vi "Main_19a.vi"() -> ()   [LabVIEW 2023]
uses:
  Cluster_Rule.ctl
  ENUM_Compare.ctl
  ENUM_Value Type.ctl
  <vilib>/Utility/error.llb/Trim Whitespace One-Sided.vi
panel:
  out "Accept Array":i32[][](array[numeric])
  out "Number Array":i32[][](array[numeric])
  out "Map":map{string, T1[]}(c390)
  out "Answer":i32
  in  "Puzzle":string="jtx{s<3181:R,R}\nrkd{s>2386:tdr,R}\nsvj{x>1520:A,A}\nvkv{x<3627:A,x>3794:A,A}\nksz{m<1450:R,a<2837:R,a<2928:R,A}\nfp{x<1293:sjt,bv}\njq{m>1493:R,m>1377:A,m<1344:R,R}\ngts{m<3166:R,A}\nxxr{s<231:R,x<3055:R,R}\nrz{a<2982:A,m<1763:R,x>1878:A,A}\nkq{s<2900:R,s>3591:A,R}\ntmg{s<1500:A,x>2504:R,a<1166:A,R}\ndvn{s<1632:R,A}\nznj{m>1884:A,R}\ndb{m<1554:cg,m>3173:R,x<1203:A,xsm}\nchr{a<682:R,x>3120:R,m>2313:A,R}\npd{x<1433:kp,a<2715:fjd,xtx}\nqkd{s<666:R,R}\nrbf{x>2541:R,R}\ngx{s>1347:A,m<812:gxz,s>1079:tpg,lt}\nfqb{x<1290:A,R}\njf{x<1340:A,s>2972:dq,x>1378:bqh,jps}\nsr{m>776:A,A}\nvs{s<1377:R,R}\nvx{x>1237:R,A}\ndz{m<192:A,m<271:A,R}\nmhr{m<2568:R,m<3466:R,a>3791:A,R}\nvv{m<3559:A,s>3108:R,R}\npsk{a>2830:A,a<2278:A,A}\ngvv{a>2993:A,a>2553:A,R}\ngsx{x<2656:A,A}\njps{a<1216:A,R}\nlt{s<967:A,A}\nng{s<3259:R,s<3674:R,A}\nzd{s>2267:R,R}\nks{a>1951:bg,m<1522:gpf,gj}\nprk{m<2242:R,s>56:R,R}\nnr{x>3432:R,sg}\nfkd{s>2014:mxf,sps}\ntk{x<1133:jzj,vq}\nsgl{a<1237:R,A}\nsmg{x<2071:R,m<387:R,A}\nqd{s<3197:sl,x>1479:lqs,m>1300:rrp,gm}\ntr{s<1306:R,x>1183:A,A}\nbxh{a>1123:fpp,R}\nhjp{a>2545:nb,a>2381:qx,m>2463:nn,bt}\nzg{s<1932:smc,m<1443:rq,jf}\nnnq{m>3341:lx,s<2737:A,a<3408:A,R}\nlx{s>3219:A,a>2886:A,m<3691:A,R}\nstl{s<2701:R,m>3442:A,s<3282:A,A}\ngsp{m<619:R,s<529:R,A}\nfkk{x<3359:svx,sp}\ndsk{x<1499:kn,xj}\njmx{m<1426:zq,fvz}\nst{s>2257:slt,rvv}\nprm{a<470:A,tts}\nfkj{x<2514:R,x>2784:R,a>2830:R,qft}\nbh{m<1740:mmf,a>503:zn,s>1702:vfp,fft}\nrv{m<2642:A,sfv}\nqk{s<1846:A,A}\nnqr{a>786:ssx,qbh}\nkng{a<3059:A,a<3463:A,a<3661:A,A}\ntcd{m<3753:R,a<2566:pq,m<3792:R,hsq}\nrhc{x>1415:mzt,x>1395:qp,x>1386:rk,nnq}\nhn{x>3532:A,a>1227:R,a>1109:A,R}\nbtd{s<2462:ftz,A}\nxv{s>1573:pv,m>730:pn,s<1201:vtz,fjk}\nsm{a>787:R,R}\nmqz{m<645:R,m<682:A,A}\nrvv{m<867:vkv,a>556:R,mx}\nfft{x>581:jb,a<314:R,R}\ntxz{s<1338:R,x>2633:A,m<1168:A,A}\npcq{x<1531:A,R}\nkvj{s<2721:A,x>2637:A,R}\nkfj{x<1129:kz,s>1501:zfm,pk}\nrd{m<3742:A,A}\nqft{x<2653:A,s>1281:A,A}\nzzr{a<3875:R,m>249:A,a<3917:R,A}\nnh{a>3744:zcn,gxg}\nfsp{m>3306:R,R}\nrt{m<310:zlk,qgj}\nmpb{m>2954:R,R}\nqgj{s>1083:R,m<502:A,s<949:A,A}\nhq{x<1527:dfg,m>3017:jvm,a>947:jts,gqf}\nbfc{x>1423:R,a<2789:A,A}\nbnv{a>900:R,A}\ntdr{a>518:R,m>657:A,x>2576:R,R}\njmm{a<3410:mq,fv}\nqjr{a>2534:R,s<1365:A,m<261:A,R}\nin{x<1624:zsf,ks}\njgs{m<702:R,A}\nqg{a<1733:A,R}\npv{x<1559:hnp,x>1588:gbv,R}\nrpx{m<2361:zv,A}\nbzm{x<1510:rhc,x<1580:lct,m>3357:rrj,zld}\ndnf{x>2931:xkp,s>1747:A,s<858:qhb,zf}\nsk{x>3528:A,x<3113:bnx,psk}\nxgt{s>2544:vn,sft}\nkjv{s>1334:gsh,a>95:rbf,a>50:bmf,trd}\npvt{s>2784:A,s<2303:qk,a<1589:A,R}\nnv{a>3108:R,x>1923:R,s>652:A,A}\nnlg{m>383:A,s>1520:A,s>749:R,R}\nlk{a<2425:R,s>598:R,a>2517:R,A}\nnt{m>1682:R,m>999:A,m>428:A,A}\nrmp{m>2634:R,s<317:nt,lk}\nfs{m<2408:A,x<1842:R,R}\nsjt{x<1133:nqr,vt}\ntbk{m<2779:R,a>3554:R,a>3415:A,R}\njr{m>3312:A,R}\nbmf{s<509:xxs,a<68:qxr,R}\nxz{s<1845:A,x<1392:A,A}\ntpn{m>2419:A,x>2999:A,s<2347:A,R}\nfcg{a<196:A,m>1248:nbt,a>276:R,R}\nkv{x>1467:R,m>891:R,s>2429:A,A}\nrq{m>570:bft,x<1349:R,m<215:R,A}\ncpr{s>140:cdl,m<2079:znj,prk}\nfc{a<3507:R,x<1454:A,s<1296:A,A}\nkfs{x<2459:R,A}\nvr{m<3596:A,a<2837:R,A}\nvg{a>3513:xl,x<569:sr,x>740:bp,qxs}\nmzc{m<3026:R,a>1169:A,A}\njhk{m<3520:A,m<3692:A,a<701:R,A}\nqx{s<1241:A,A}\nbv{x<1412:zg,m<1721:hh,hq}\npj{s>3641:A,x>1535:mj,m<1145:A,jxb}\nsvx{x<3194:A,m<1734:gsp,m<2937:zk,kng}\nkp{x<1404:jj,m>1015:R,x>1415:bfc,A}\ncxh{m>619:R,m>536:A,R}\nffj{x<2728:R,s<231:A,R}\nfh{m<1629:A,a<1260:A,A}\ntrd{a>29:qc,A}\nhj{a<706:kvj,s<3197:grd,a>1057:mzc,gsx}\nqcx{a<265:R,R}\nbhz{x<1415:R,A}\nccq{a<3195:mtr,a<3700:jzv,x>1501:xv,tj}\nqpn{s>499:vpz,a>804:qsc,lsm}\njk{x<3497:R,x>3734:A,A}\nbz{x>568:A,a<773:A,R}\nhkv{a<1753:R,x<2544:A,a>1849:R,ps}\ngj{m>2405:fkd,s>1405:pf,qpn}\nlg{a<1611:rlx,a<1731:fps,A}\nln{a<1637:R,s<3175:A,A}\nshk{a<1729:htt,m>1833:R,A}\nsct{m>1497:A,R}\nrnj{a>2878:R,m>1475:R,a<2792:R,A}\nqp{a<3308:R,m>3268:vv,A}\nvq{s<2622:R,R}\nnbt{s<1656:A,m<1413:R,m>1485:A,A}\nbdm{x<2476:gv,x>2650:vhv,kh}\nbjh{x<2660:R,A}\nfnx{a<3874:A,A}\nqzt{s>3620:A,A}\nft{a<1286:A,m>1846:R,R}\ncx{a>2841:A,m<425:qjr,s>1229:qm,R}\nrrj{m<3695:nm,m>3867:sz,a>3080:cd,tcd}\nghj{s<2416:A,m<2698:R,R}\nxm{a<3638:pcq,m>2433:pnx,tsc}\nhkg{a<1186:A,R}\nts{s>905:A,m<299:R,R}\ndbf{m<1691:sct,s<3740:mnr,A}\nssq{s>3183:A,m<2388:A,A}\nbd{s>291:jbg,s<217:R,s<250:ffj,vl}\ndq{a<1136:R,R}\nrpf{s>2706:ll,x<2910:ghj,A}\nqxr{s<877:A,A}\nlct{s>3272:kx,hcp}\nbbc{a<3031:R,x<1554:A,R}\nzlk{m>176:R,A}\nlh{a<3217:fld,x<504:jr,rgg}\nzct{x>2738:sk,x>2209:bdm,gdm}\ndj{x>1137:A,a>2578:A,R}\ngc{a>2861:R,a<2739:A,A}\nlhn{s>2175:jz,m>1213:hcq,lxj}\nqm{x<1501:R,s>1724:R,A}\nbnx{s>3556:R,x<2924:A,a>2767:A,R}\nzr{s<2643:A,ms}\nsmc{x<1354:R,x>1374:R,s>1279:fh,cxb}\njvm{s>1609:zmn,a<1172:jhk,cxl}\nsz{s>3310:A,R}\nbxf{a>2995:A,rnj}\nqn{x>1577:A,R}\nrm{x>3502:sm,x<3166:rzf,R}\nzzd{a<2945:A,s<530:A,a<3360:A,A}\nns{x<1515:A,a<2501:A,R}\nrnb{s<1360:A,m>2498:R,s<1805:R,A}\nsrj{x>1408:R,R}\njzv{m>750:ltd,s<1511:rt,tcc}\ngps{a>3444:A,x>1039:R,x<989:R,A}\ncmr{x<2302:A,R}\nmgq{a>3431:A,m<2513:R,R}\nzps{m<2495:R,x>1582:A,a>3314:R,A}\nxj{s<2468:A,x>1516:A,a>3292:A,A}\nhfv{a>2835:phz,x<1072:jc,dj}\nvmf{a<2879:qdv,m<1506:xsn,x>2082:rr,xdq}\nndj{m>605:A,a>1367:R,A}\nsd{x>1431:A,a<3334:A,s>3667:A,A}\nfjt{a<2589:R,A}\nslp{x<583:A,A}\njfx{s>639:R,s>549:R,zc}\nzrc{m<2490:A,fsp}\nsqf{s>3315:A,m<2054:A,R}\nhlm{a<3112:R,m>1347:A,R}\nbp{s>2210:A,R}\nhtt{a<1620:R,R}\nlhg{x>1534:rb,m>1305:qmz,a>2889:dsk,rs}\ncxl{a<1794:R,a<2060:R,m>3613:R,R}\nlrt{x>1214:A,m<826:A,x<1148:R,A}\nkdt{a>3422:A,a>3354:vx,a<3313:A,ff}\nqc{s>566:R,a<43:R,A}\njnn{s>1664:zsx,m<3370:tmg,m<3740:R,lj}\nrlx{s>2568:A,s>1841:R,x<2496:A,R}\ncxb{x>1364:R,A}\nvp{m<625:mt,m>1209:psm,prx}\njbz{x<1581:A,R}\nfld{x>580:A,a<2939:vz,qt}\ngz{m<2078:A,m>2102:A,m>2086:R,A}\npq{s<3162:R,s<3713:R,R}\nnvr{a>3064:R,x>1573:A,a>2695:R,A}\nmt{m<212:xgt,m<391:msk,a<1427:dh,nqj}\nqq{m<1871:A,x>2374:A,m>2819:R,R}\nkx{s>3712:R,a<3138:A,a>3552:A,sb}\nzl{a<3279:R,s>3644:R,s<3369:R,A}\nzhr{x>1414:mhr,s<1315:R,R}\nlr{a<3472:fl,x<1240:qzt,m>1702:A,A}\nzn{m>3032:bz,R}\nkdb{m>2017:lh,vg}\nxdq{a>3298:fs,s>454:nv,R}\njj{x<1385:R,s>2524:A,a<2778:R,R}\nhh{s>1624:bqx,m<725:lf,m<1340:hkg,qkd}\ntt{x>3601:A,R}\nff{m>2244:A,x>1175:R,s>652:A,A}\nnb{m<2342:sx,s<1466:A,gc}\ngg{x>2442:R,A}\nzf{x>2749:A,R}\nms{a<3730:A,A}\npnx{a>3878:A,R}\nthm{a<2994:R,m<2863:R,R}\ndcn{x<1937:R,x>2071:A,m<1510:R,R}\nzh{x<1391:A,a<2729:A,R}\nmzt{m>3358:R,s>2801:thm,x>1477:kzl,A}\nvk{x<1245:hfv,a<2636:rmp,ldb}\ncdl{x>2787:A,A}\ngsh{x>2372:A,s<2731:tgk,ng}\nss{s>1887:A,R}\nlsm{a<346:qqd,s<179:pls,a<518:hxk,bd}\nkl{m<767:cm,s>2943:hlm,s<2861:R,R}\njc{a>2461:R,R}\nlq{x<3091:A,m>3019:R,s<338:R,A}\ndc{m>3120:R,s<2936:R,A}\nfjx{a<3729:R,m>577:bhz,A}\nslh{s<2472:A,x>841:A,x>782:A,R}\njn{a>3008:A,m<154:R,A}\nrnt{m<1544:fqb,pt}\nlzl{a>2640:kk,s<3306:A,x<1073:R,kft}\nrjm{a<2579:R,x<1122:A,x<1178:A,A}\nxxn{a>3097:R,x>2616:R,x>2520:A,R}\ngmk{a>432:rkd,m<699:mp,np}\ngk{a<343:xnh,st}\nmtr{m<974:cx,a>2634:lp,a>2480:mb,vvl}\nsn{s<1735:R,x>3011:R,A}\nhcp{m<2836:A,A}\nbzv{m<2882:A,m>3102:A,x>1615:A,R}\ngpf{a>786:vp,x>3204:gk,fgh}\nbqh{x>1390:A,a<781:A,a<1479:R,A}\nzk{s<581:R,a>3168:R,A}\nrzf{x>2996:R,A}\npt{m>2840:R,sqf}\ndr{a<1633:R,rx}\nbj{m<2330:A,R}\nrp{a<2416:A,x<1528:A,R}\nfv{x<1478:zhr,xm}\nzkq{s>2684:zct,jmx}\nhg{x>1427:xkb,s>2386:R,s>2348:jgs,R}\nljp{x<3070:qmk,vkc}\nqcd{x>2958:kq,m<1982:R,A}\ndh{a<1030:A,x<2896:tns,s>1349:hn,A}\nnn{a<2330:A,s<1631:A,x>1119:R,A}\ntcc{x<1454:xz,s>1712:xb,x>1524:dvn,tb}\nprd{m>3593:R,s<3539:A,A}\nprx{s<1392:pm,a<1410:bxh,lg}\ndnj{s>2561:zr,m>1174:nh,s<2439:hg,fjx}\nltr{s<2819:chr,x>3007:fmv,ndx}\nzls{s<2833:R,x>2257:R,R}\ntj{a>3851:bfb,gx}\ncqn{x>1072:rjm,s<3160:ktb,fjt}\nsps{a<845:gts,a>1373:hkv,s>1282:jnn,mcd}\npk{x>1234:A,s>1197:tr,x<1173:cl,R}\nlp{a>3002:R,s>1470:R,m<1336:A,ksz}\nbnl{a<1615:A,s<1889:R,a<2234:R,R}\npx{x>2650:ln,m>3593:A,zls}\nbqx{m<671:zvx,m>1076:A,x>1511:R,kv}\ntg{x<1547:R,a>3186:A,a<2861:R,A}\nbbv{x>1046:A,R}\nnl{m>2498:A,s<1270:R,s>1844:R,R}\ngxg{a<3560:A,A}\nhtm{a>1548:R,ft}\njzj{a<3414:R,s>2535:R,a<3803:A,R}\ntl{m>591:R,s<2128:R,A}\nlj{a>1135:R,A}\nqt{x>217:A,a>3101:A,R}\nzmn{x>1568:R,m<3662:A,s>2942:R,A}\ngqf{a<319:A,lc}\npn{x<1566:fnx,R}\nlm{x<748:A,m>1097:slh,mnc}\nxb{a>3483:A,R}\nhbn{x<2347:rz,s<1021:xxn,bj}\nfps{s<2809:R,m>978:R,a<1677:R,A}\ntns{m>508:A,R}\nftz{m<1047:A,R}\nhsq{s<3306:A,R}\nrcf{m<789:R,a>3811:A,R}\nzsx{m<3362:A,A}\nqnm{m<1707:jq,m>1918:A,klh}\nktb{a>2476:R,a<2324:R,m<1618:R,R}\ntts{s<974:A,a>655:R,x>2433:A,A}\nnf{a<3288:vk,zpd}\ncj{x<1368:dll,m>2179:bzm,s<2729:ntm,qd}\nvtz{s>967:zzr,x<1579:R,ts}\nzv{a>3078:R,A}\nxxs{a>80:R,m<655:R,A}\ntsc{a<3864:A,a>3938:R,m>1924:R,R}\nbf{x>2895:fkk,vmf}\nrk{m>3266:R,m>2870:dc,a<3009:zh,mgq}\nnqj{s>1829:R,s>913:vs,mnk}\nfd{s<871:A,R}\nmj{m>871:A,a>2639:R,a<2371:A,A}\nqbm{m>1109:A,s>3601:R,x>1512:R,A}\ndpc{m<2093:sgl,R}\nvkc{a>3311:ghs,a>2714:bxf,rv}\nsx{s>1313:R,A}\ngl{x>1498:qbm,m<1020:rg,A}\njbx{a>706:R,x>2598:A,pb}\nhxk{a>436:tgn,gs}\ntpg{s>1250:R,m>1185:A,s<1173:A,R}\nqdv{s<616:mkj,qq}\nmsk{a<1506:sn,s>2324:A,qg}\nxjk{s>2290:R,R}\ngrd{s<2548:R,A}\nxlg{s>3562:A,a>543:A,A}\nxnh{x<3580:nr,m>777:fcg,m<313:vpk,vbp}\nkh{m<1498:A,A}\nzsf{x<948:mf,a<2235:fp,s>2045:cj,zhj}\nxsm{s<799:R,x<1241:R,a>872:A,R}\nxp{m<1016:R,R}\nvpk{x<3813:tv,R}\nrr{s<604:R,R}\nslt{s<3054:tt,s>3473:A,R}\npxn{m<2918:R,R}\ntqg{m>2713:gvv,x<1585:zps,A}\nxl{a<3724:R,m<814:A,m<1249:R,R}\nlqs{a<3226:pj,x<1533:gl,a>3574:nqz,cnm}\nqhb{m>398:R,s>521:A,x<2791:A,R}\npp{a>3287:A,s<2490:R,a<3039:A,A}\nklh{a>3097:A,a<2627:A,x>1416:A,R}\nkzl{x>1498:A,R}\ncd{m>3789:R,s>2774:rd,jjh}\nqvj{s>2916:lb,m>1773:gg,A}\nnm{m<3503:stl,a>3204:jtx,s<3198:vr,prd}\nzfm{a<3405:cf,x>1270:dk,A}\ndll{a>2858:kr,x<1210:cq,rnt}\nzvx{m<440:A,R}\nrs{s>2487:A,m>583:A,m<352:zvt,ns}\ngv{x>2386:A,x<2306:A,A}\ntsg{x>1593:R,A}\nbft{m<1111:R,A}\nzld{x<1595:tqg,a<3278:pxn,ds}\nnlj{s<37:A,R}\ndd{m<360:jn,x<1406:xlx,zl}\nxkp{a>723:R,a>685:A,a>649:A,A}\nphz{a>3010:R,R}\nzvv{m>587:btd,m<276:jbx,x>2637:dnf,smg}\nldb{s>500:R,s<176:A,x>1432:svj,sv}\ngm{m<544:dd,sd}\nrrp{s>3471:dbf,qnm}\ntgk{s>1833:R,m>698:A,a<170:A,A}\ntf{a<2989:R,s<2648:R,m<978:A,A}\njv{a>1049:bk,bh}\nzjq{x<394:A,s<2172:A,x>409:R,A}\nsb{a>3392:A,s<3499:A,s<3590:A,A}\ngbv{s>1783:R,m<518:A,R}\nmb{a<2566:R,A}\njbg{x<2977:A,R}\ncq{m>2591:lzl,cqn}\ngpp{s>127:A,R}\nqxs{x<630:R,R}\nltd{m<1040:fc,s<1339:R,fzh}\ntv{m<191:R,R}\nvbp{m>508:A,a<198:hc,m<391:R,qcx}\nqhx{s<1393:A,A}\nzt{x<829:A,s>2272:A,m>3119:R,A}\nxlx{s<3549:R,s<3703:R,a<2825:A,A}\nmnc{m>410:R,x<820:R,A}\njts{s>2528:A,a>1459:A,nl}\nvfp{a<268:slp,a<349:A,A}\nxkb{s>2400:A,a>3661:R,s<2364:A,R}\njxb{x>1512:R,m>1668:R,s<3371:R,A}\njjh{s>2302:A,s<2157:R,R}\ndfg{m<3080:bnv,R}\nsft{m>85:R,A}\nkft{s<3765:R,x<1151:A,A}\nql{m<2989:bnl,A}\nhmq{s>328:A,R}\nzgl{s<3038:xp,s>3136:R,tg}\njz{x<1535:nz,vcx}\nfpp{a<1269:A,s<2540:R,m<877:A,A}\nsl{x<1465:kl,zgl}\nghs{s<1180:jk,A}\ngdm{s<3410:A,dcn}\nmp{a>355:nlg,x>2257:A,R}\ntgn{s>384:A,A}\nrck{a>3096:A,m<729:R,R}\nbfh{s<2430:A,A}\ndm{x<3740:A,a<84:A,R}\ncl{x>1152:A,a>3659:A,A}\nlf{s<590:A,m<384:dz,ndj}\nkr{s<3089:tk,x>1116:lr,fq}\nps{x<3131:R,a>1808:R,R}\nzc{a<3742:R,s<459:A,A}\nhdq{a>1180:A,a<969:A,m<1327:xjk,vxc}\nvtn{x>2571:gz,A}\nvsp{m<1477:kf,m>1506:A,x<1988:A,R}\npf{m<1916:zj,nsl}\nqqb{a<3381:R,a<3544:A,R}\nqmk{s>1137:fkj,hbn}\nfjk{m<484:qhx,s>1346:mqz,a<3843:qn,cxh}\nfzh{a>3465:R,s<1753:A,R}\nll{a<1599:A,m>2800:R,m<2548:R,R}\npm{x<2958:A,A}\nds{s>3322:A,x>1607:bzv,s<2559:A,tbk}\nqqd{a>147:xxr,x<2716:hmq,x<3308:R,dm}\nzj{x>2856:rm,a>694:qvj,jkr}\nntm{s<2328:lhn,x>1477:lhg,a<3351:pd,dnj}\ngs{x>3009:R,m>1822:R,m>1623:A,A}\nvpz{a<955:prm,htm}\nfl{s<3647:A,R}\nvf{m>1405:R,x<364:R,x<439:zjq,A}\nsfv{m>3249:R,a<2323:A,a<2508:A,R}\nssx{s<1450:R,R}\nxtx{s<2531:bfh,tf}\nfvz{s<1875:R,a<2683:tpn,s<2272:kfs,pp}\nzpd{s<374:gpp,a<3568:kdt,jfx}\nbq{a>2468:A,R}\nmx{x>3691:R,A}\nzvt{m<232:R,x<1498:R,R}\nqbh{a>359:bbv,A}\nrx{s<1895:R,x<93:A,R}\npls{s<102:nlj,m>1957:A,x>2610:R,R}\ngxz{x<1441:A,a>3782:A,a<3736:A,A}\nvcx{x<1581:A,x>1598:R,A}\nmnk{x>2686:R,A}\nhc{m>386:R,s<1896:R,x>3841:A,R}\njkr{x<2289:R,a<434:bjh,s>2706:xlg,ddr}\nlxj{x<1526:A,a<2868:tl,s<2105:A,R}\ncs{s>2587:A,s<2454:R,x>1605:A,A}\ntb{a<3403:R,x<1483:A,m<408:A,R}\njrk{x<1493:R,A}\nnp{s<2392:txz,R}\nfgh{a<278:kjv,a>610:zvv,gmk}\nnsl{a>1286:pvt,m>2128:ltr,m<2048:qcd,vtn}\nsp{x<3783:zzd,R}\nmnr{a<2963:R,R}\nkn{s>2492:R,R}\nsg{x>3309:R,A}\nkf{x>1948:A,A}\nsv{x>1311:A,m>2072:A,R}\nddr{a>588:R,A}\nmmf{s>1614:A,a<588:fd,s>637:A,R}\nmzd{a>3041:kfj,hjp}\njb{x>749:A,x<663:R,a<217:R,A}\nzq{x<2680:rck,zd}\nkk{s>3062:A,x<1054:R,x>1150:R,A}\nmcd{s>737:R,lq}\nkm{a<454:ssq,x>1215:A,R}\njp{m>1384:R,a>1361:A,m<1302:R,A}\nzcn{m>1641:A,x<1412:R,a<3907:R,R}\nhnp{m<624:R,m<1118:R,a>3867:A,A}\nvvl{a>2360:jrk,A}\nvt{a>1209:zrc,s>2239:km,a>526:db,rnb}\nxsn{a<3485:A,x>2424:rcf,x<2143:R,cmr}\nfmv{m>2241:A,A}\nmq{a<2726:rp,rpx}\nqsc{a>1561:shk,s>289:dpc,cpr}\nvn{x<2495:A,R}\nzhj{s<820:nf,x<1349:mzd,m<1523:ccq,jmm}\nrb{x>1585:cs,x<1567:bbc,m>1281:nvr,R}\nvl{a<701:A,a<749:R,R}\nbk{m>2181:ql,x>534:lm,x>246:vf,dr}\nbt{s<1575:R,x>1110:lrt,A}\ncg{x<1226:R,R}\npb{s>1976:R,R}\nqmz{x>1511:R,hx}\nhx{s<2479:A,a>3026:R,x>1492:A,R}\nvxc{s<1908:R,R}\npsm{x>2500:vmq,m<1395:hdq,vsp}\nbg{s>1448:zkq,s<952:bf,ljp}\nrg{a<3524:R,R}\nmxf{a<1247:hj,m<3013:rpf,px}\ncnm{m<854:A,s>3702:A,A}\nfjd{m>911:A,s>2513:bq,A}\nmkj{x>2290:R,m<1691:A,s>347:A,A}\nvhv{s>3440:A,x<2695:R,R}\nhcq{a>2835:R,R}\nvmq{s>2256:A,s<1332:jp,x<3237:ss,A}\nnz{a<3118:A,x<1466:R,s<2259:A,R}\nndx{m>2236:R,x>2459:A,s<3532:R,A}\nkz{s<1342:R,R}\nlb{s>3471:A,a>1457:A,A}\nvz{a>2782:R,A}\ncm{a<3264:R,a>3609:R,A}\nnqz{s>3591:R,m>1381:jbz,m<596:A,tsg}\ndk{x<1297:A,a>3642:R,A}\nmf{a<2621:jv,kdb}\nlc{x<1574:A,m>2523:R,a<541:A,A}\ncf{a<3177:R,R}\nrgg{x>754:zt,a<3650:qqb,mpb}\nfq{s<3534:R,s<3736:gps,R}\nbfb{s>1404:R,s>1128:R,srj}\n\n{x=61,m=577,a=1750,s=1892}\n{x=8,m=603,a=567,s=987}\n{x=1398,m=1265,a=702,s=949}\n{x=2322,m=693,a=2401,s=946}\n{x=348,m=2812,a=613,s=1788}\n{x=3353,m=2070,a=1617,s=3088}\n{x=24,m=963,a=4,s=1053}\n{x=396,m=877,a=3375,s=127}\n{x=1490,m=100,a=1060,s=724}\n{x=413,m=95,a=944,s=847}\n{x=1580,m=960,a=880,s=1400}\n{x=1956,m=597,a=3294,s=284}\n{x=1924,m=21,a=726,s=1276}\n{x=1338,m=1630,a=348,s=114}\n{x=11,m=1649,a=475,s=1091}\n{x=1660,m=563,a=1047,s=150}\n{x=18,m=226,a=33,s=3744}\n{x=3145,m=482,a=866,s=629}\n{x=474,m=260,a=1408,s=9}\n{x=361,m=1348,a=592,s=380}\n{x=2632,m=1281,a=234,s=1114}\n{x=1871,m=543,a=1285,s=383}\n{x=1870,m=364,a=106,s=70}\n{x=536,m=528,a=272,s=2050}\n{x=1519,m=1564,a=434,s=103}\n{x=301,m=2005,a=1069,s=79}\n{x=293,m=143,a=3201,s=68}\n{x=1308,m=1701,a=271,s=1627}\n{x=1538,m=1576,a=249,s=290}\n{x=320,m=110,a=1490,s=492}\n{x=494,m=904,a=2049,s=1122}\n{x=13,m=695,a=1851,s=145}\n{x=136,m=1102,a=90,s=879}\n{x=1786,m=8,a=663,s=86}\n{x=238,m=2582,a=1288,s=3169}\n{x=1628,m=1807,a=373,s=116}\n{x=86,m=51,a=500,s=1893}\n{x=2848,m=36,a=2897,s=1757}\n{x=774,m=530,a=970,s=2379}\n{x=353,m=1490,a=844,s=2085}\n{x=1363,m=938,a=1103,s=1200}\n{x=1843,m=6,a=1853,s=882}\n{x=1966,m=3149,a=327,s=201}\n{x=1116,m=849,a=1822,s=326}\n{x=233,m=3172,a=32,s=1141}\n{x=3523,m=19,a=38,s=176}\n{x=2896,m=511,a=1180,s=2859}\n{x=292,m=843,a=98,s=98}\n{x=923,m=606,a=2898,s=2343}\n{x=46,m=1317,a=78,s=51}\n{x=462,m=1255,a=1485,s=737}\n{x=1238,m=1292,a=27,s=1525}\n{x=2731,m=411,a=1831,s=1574}\n{x=202,m=426,a=483,s=349}\n{x=33,m=394,a=941,s=1705}\n{x=2648,m=510,a=703,s=2332}\n{x=1429,m=836,a=316,s=63}\n{x=2817,m=1701,a=174,s=160}\n{x=261,m=206,a=76,s=2192}\n{x=204,m=2989,a=283,s=597}\n{x=1068,m=1881,a=3293,s=2503}\n{x=31,m=37,a=826,s=2983}\n{x=547,m=466,a=1586,s=481}\n{x=1419,m=822,a=273,s=1670}\n{x=392,m=168,a=452,s=61}\n{x=1245,m=2719,a=778,s=2034}\n{x=1150,m=1565,a=1098,s=502}\n{x=1180,m=30,a=1228,s=223}\n{x=727,m=6,a=224,s=144}\n{x=1784,m=863,a=741,s=1461}\n{x=1200,m=1331,a=113,s=1114}\n{x=3108,m=312,a=246,s=1943}\n{x=970,m=1845,a=3752,s=940}\n{x=2062,m=420,a=290,s=264}\n{x=1626,m=1844,a=337,s=321}\n{x=1124,m=1302,a=335,s=1250}\n{x=205,m=203,a=102,s=292}\n{x=228,m=1798,a=562,s=326}\n{x=897,m=832,a=1193,s=1826}\n{x=336,m=1941,a=1348,s=2270}\n{x=162,m=275,a=3043,s=1022}\n{x=361,m=268,a=2199,s=1749}\n{x=328,m=1482,a=1865,s=1420}\n{x=474,m=2434,a=2447,s=1199}\n{x=1066,m=3051,a=1482,s=50}\n{x=252,m=1317,a=349,s=894}\n{x=1241,m=283,a=3431,s=503}\n{x=958,m=403,a=928,s=487}\n{x=1193,m=830,a=3266,s=2617}\n{x=914,m=1239,a=275,s=3325}\n{x=2885,m=1206,a=1998,s=313}\n{x=831,m=1327,a=447,s=181}\n{x=3912,m=2397,a=522,s=1136}\n{x=2222,m=375,a=1129,s=595}\n{x=3340,m=205,a=1197,s=1910}\n{x=2206,m=20,a=1354,s=63}\n{x=1068,m=916,a=10,s=1564}\n{x=316,m=827,a=371,s=1808}\n{x=3287,m=329,a=2730,s=22}\n{x=863,m=2792,a=321,s=1546}\n{x=1470,m=301,a=795,s=249}\n{x=582,m=96,a=2814,s=1126}\n{x=387,m=461,a=1526,s=355}\n{x=23,m=1590,a=1448,s=269}\n{x=1983,m=165,a=714,s=1140}\n{x=513,m=1006,a=835,s=1438}\n{x=25,m=280,a=1263,s=2950}\n{x=823,m=973,a=949,s=166}\n{x=720,m=255,a=92,s=184}\n{x=867,m=1262,a=153,s=569}\n{x=443,m=376,a=4,s=656}\n{x=108,m=600,a=958,s=64}\n{x=609,m=1212,a=3436,s=1060}\n{x=267,m=645,a=2807,s=959}\n{x=159,m=2,a=557,s=1673}\n{x=2744,m=49,a=49,s=2043}\n{x=835,m=33,a=1119,s=440}\n{x=2697,m=499,a=386,s=1553}\n{x=456,m=110,a=666,s=625}\n{x=1274,m=1335,a=336,s=124}\n{x=2341,m=1835,a=100,s=2163}\n{x=2104,m=1161,a=234,s=1831}\n{x=915,m=1660,a=792,s=429}\n{x=314,m=384,a=33,s=294}\n{x=628,m=579,a=2605,s=1746}\n{x=2,m=2227,a=1151,s=38}\n{x=294,m=1196,a=1330,s=295}\n{x=517,m=2634,a=994,s=267}\n{x=272,m=25,a=882,s=217}\n{x=599,m=652,a=951,s=126}\n{x=255,m=650,a=955,s=102}\n{x=25,m=1704,a=2216,s=13}\n{x=142,m=817,a=208,s=921}\n{x=1932,m=746,a=1646,s=2252}\n{x=1157,m=6,a=2213,s=3366}\n{x=595,m=10,a=2,s=2750}\n{x=696,m=955,a=3215,s=8}\n{x=2223,m=3582,a=47,s=1055}\n{x=302,m=330,a=420,s=495}\n{x=128,m=2241,a=1155,s=387}\n{x=225,m=151,a=682,s=916}\n{x=844,m=181,a=1842,s=2310}\n{x=270,m=837,a=1311,s=2122}\n{x=3135,m=829,a=1974,s=164}\n{x=1061,m=1019,a=2238,s=571}\n{x=2109,m=1065,a=316,s=1054}\n{x=1523,m=512,a=42,s=342}\n{x=1378,m=2105,a=1968,s=3674}\n{x=51,m=94,a=683,s=832}\n{x=235,m=1036,a=121,s=741}\n{x=18,m=713,a=250,s=484}\n{x=193,m=2650,a=569,s=210}\n{x=1203,m=2854,a=644,s=515}\n{x=3,m=881,a=967,s=1500}\n{x=375,m=2028,a=214,s=135}\n{x=1693,m=696,a=2186,s=138}\n{x=1347,m=655,a=722,s=111}\n{x=678,m=995,a=3274,s=183}\n{x=1720,m=242,a=1637,s=933}\n{x=798,m=1710,a=3735,s=1521}\n{x=3046,m=335,a=1055,s=296}\n{x=632,m=6,a=207,s=591}\n{x=109,m=2344,a=40,s=413}\n{x=387,m=121,a=171,s=2554}\n{x=1546,m=159,a=2373,s=1578}\n{x=875,m=21,a=377,s=2524}\n{x=1641,m=1125,a=694,s=2737}\n{x=188,m=310,a=378,s=498}\n{x=589,m=174,a=2495,s=2769}\n{x=2918,m=258,a=643,s=47}\n{x=833,m=214,a=333,s=24}\n{x=1982,m=200,a=569,s=1014}\n{x=341,m=196,a=1404,s=286}\n{x=1009,m=248,a=281,s=1903}\n{x=547,m=2531,a=215,s=117}\n{x=904,m=249,a=46,s=109}\n{x=186,m=1706,a=1307,s=732}\n{x=1182,m=1615,a=299,s=1275}\n{x=2136,m=1349,a=1907,s=523}\n{x=13,m=1375,a=1617,s=1599}\n{x=786,m=131,a=541,s=67}\n{x=12,m=223,a=1565,s=129}\n{x=837,m=261,a=22,s=363}\n{x=1011,m=249,a=146,s=251}\n{x=711,m=230,a=3042,s=246}\n{x=2794,m=1052,a=243,s=457}\n{x=2289,m=1093,a=2061,s=1219}\n{x=2223,m=176,a=1227,s=444}\n{x=1744,m=37,a=1590,s=87}\n{x=2590,m=2444,a=894,s=1864}\n{x=13,m=1356,a=648,s=121}\n{x=117,m=125,a=1222,s=669}\n{x=1048,m=419,a=1031,s=210}\n{x=397,m=2126,a=412,s=977}\n{x=1256,m=875,a=3898,s=3195}\n{x=3273,m=322,a=702,s=4}\n{x=956,m=500,a=522,s=596}\n{x=339,m=1107,a=2588,s=970}\n{x=493,m=43,a=1683,s=1244}\n{x=303,m=484,a=425,s=207}"
  in  "Example":string="px{a<2006:qkq,m>2090:A,rfg}\npv{a>1716:R,A}\nlnx{m>1548:A,A}\nrfg{s<537:gd,x>2440:R,A}\nqs{s>3448:A,lnx}\nqkq{x<1416:A,crn}\ncrn{x>2662:A,R}\nin{s<1351:px,qqz}\nqqz{s>2770:qs,m<1801:hdj,R}\ngd{a>3333:R,R}\nhdj{m>838:A,pv}\n\n{x=787,m=2655,a=1222,s=2876}\n{x=1679,m=44,a=2067,s=496}\n{x=2036,m=264,a=79,s=2244}\n{x=2461,m=1339,a=466,s=291}\n{x=2127,m=1623,a=2188,s=1013}"
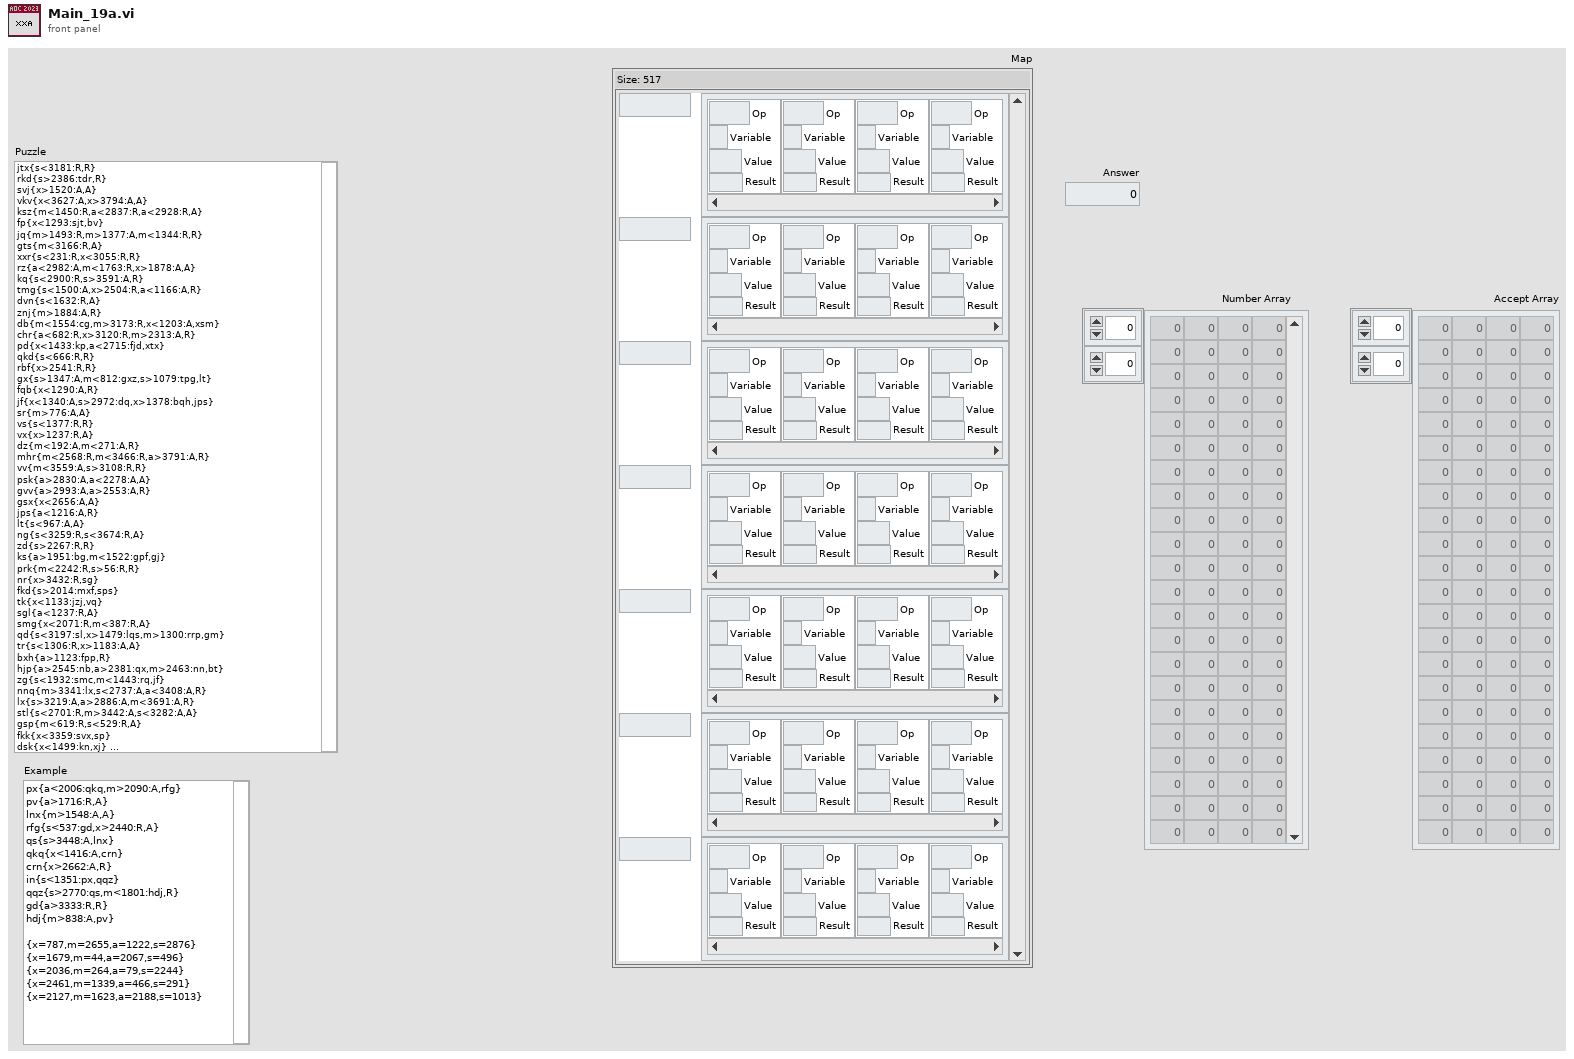
[diagram p1: front panel]
types:
  T1 = typedef "Cluster_Rule.ctl" = cluster{"Op":T2, "Variable":T3, "Value":i32, "Result":string}
  T2 = typedef "ENUM_Compare.ctl" = enum16{"TRUE", "<", ">", "<=", ">="}
  T3 = typedef "ENUM_Value Type.ctl" = enum16{"x", "m", "a", "s"}
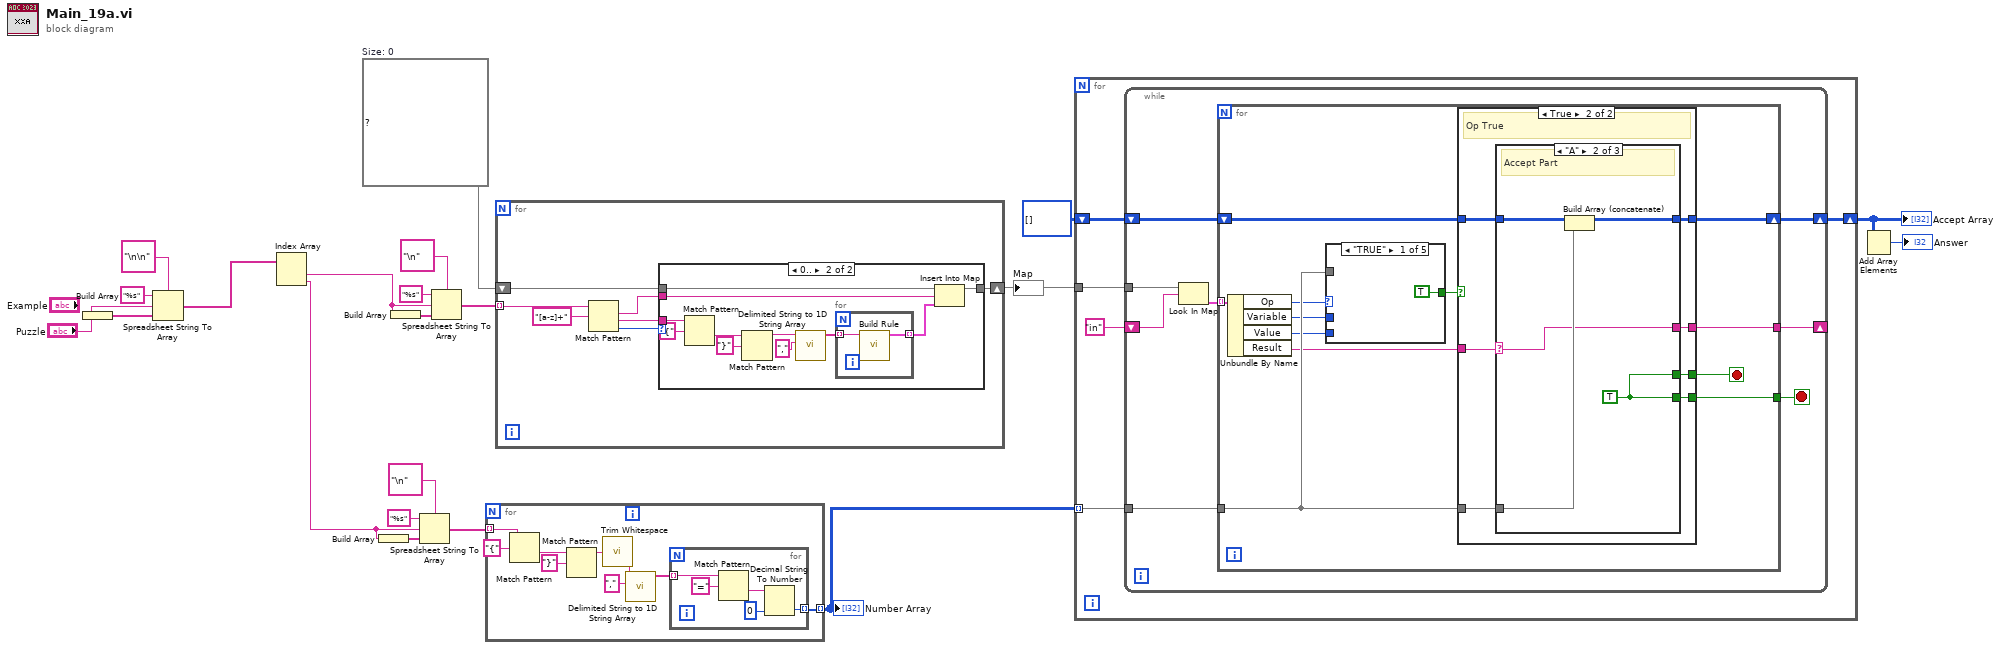
[diagram p0: block diagram]
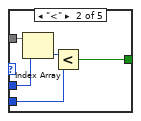
[diagram p2: hidden frame]
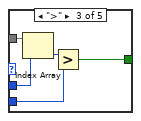
[diagram p3: hidden frame]
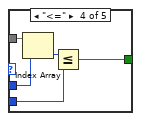
[diagram p4: hidden frame]
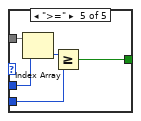
[diagram p5: hidden frame]
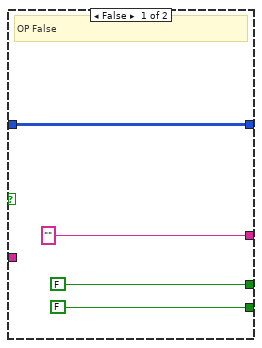
[diagram p6: hidden frame]
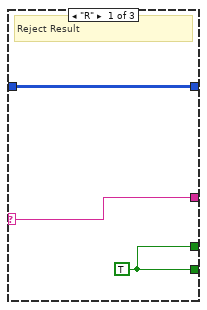
[diagram p7: hidden frame]
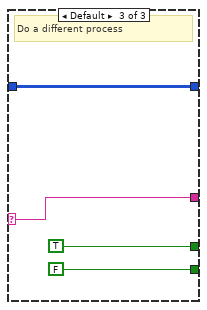
[diagram p8: hidden frame]
diagram:
  w18 = map{string, T1[]} {}  # Size: 0
  n1 = Build Array("Puzzle") -> (w21:string[])
  n2 = Spreadsheet String To Array(delimiter (Tab)="\n\n", format string="%s", spreadsheet string="Puzzle", array type (2D Dbl)=w21) -> (array=w13:string[])
  n3 = Index Array(array=w13) -> (element #1=w15:string, element #2=w8:string)  [unwired: 2 in]
  n4 = Build Array(w8) -> (w11:string[])
  n5 = Build Array(w15) -> (w14:string[])
  n6 = Spreadsheet String To Array(delimiter (Tab)="\n", format string="%s", spreadsheet string=w8, array type (2D Dbl)=w11) -> (array=w7:string[])
  n7 = Spreadsheet String To Array(delimiter (Tab)="\n", format string="%s", spreadsheet string=w15, array type (2D Dbl)=w14) -> (array=w12:string[])
  n8 = for {
    tunnel: w7 -> [w27] mode=indexing
    tunnel: [w22] -> w6 mode=indexing
    n9 = Match Pattern(string=w27, regular expression="{") -> (after substring=w29:string)  [unwired: 1 in, 3 out]
    n10 = Match Pattern(string=w29, regular expression="}") -> (before substring=w26:string)  [unwired: 1 in, 3 out]
    n11 = call <vilib>:"Trim Whitespace.vi"("string"=w26) -> ("trimmed string"=w25:string)  [unwired: 1 in]
    n12 = call <vilib>:"Delimited String to 1D String Array.vi"("delimiter"=",", "delimited string"=w25) -> ("string array"=w23:string[])  [unwired: 9 in]
    n13 = for {
      tunnel: w23 -> [w35] mode=indexing
      tunnel: [w31] -> w22 mode=indexing
      n14 = Match Pattern(string=w35, regular expression="=") -> (after substring=w33:string)  [unwired: 1 in, 3 out]
      n15 = Decimal String To Number(string=w33, default (0L)=0 ("default (0 I32)")) -> (number=w31:i32)  [unwired: 1 in, 1 out]
    }
  }
  "Number Array" <- w6
  n16 = for {
    tunnel: w12 -> [w42] mode=indexing
    shift-right: [w39] -> w5
    shift-left: w18 -> [w38]
    n17 = Match Pattern(string=w42, regular expression="[a-z]+") -> (match substring=w37:string, after substring=w40:string, offset past match=w36:i32)  [unwired: 1 in, 1 out]
    n18 = case shown="0.." w36 {
      tunnel: w40 -> [_ w54]
      tunnel: [w43 w47] -> w39
      tunnel: w38 -> [w43 w46]
      tunnel: w37 -> [_ w44]
      frame ..-1 {
      }
      frame 0.. {
        n19 = Match Pattern(string=w54, regular expression="{") -> (after substring=w52:string)  [unwired: 1 in, 3 out]
        n20 = Match Pattern(string=w52, regular expression="}") -> (before substring=w50:string)  [unwired: 1 in, 3 out]
        n21 = call <vilib>:"Delimited String to 1D String Array.vi"("delimiter"=",", "delimited string"=w50) -> ("string array"=w48:string[])  [unwired: 9 in]
        n22 = for {
          tunnel: w48 -> [w56] mode=indexing
          tunnel: [w55] -> w45 mode=indexing
          n23 = call "Build Rule.vi"("String"=w56) -> ("Cluster"=w55:T1)  [unwired: 10 in]
        }
        n24 = Insert Into Map(map in=w46, key=w44, value=w45) -> (map out=w47:map{string, T1[]})  [unwired: 2 out]
      }
    }
  }
  "Map" <- w5
  n25 = for {
    tunnel: w6 -> [w59] mode=indexing
    tunnel: w5 -> [w61]
    shift-right: [w57] -> w3
    shift-left: i32[][] [] -> [w58]
    n26 = while {
      tunnel: w61 -> [w69]
      shift-right: [w62] -> _
      shift-left: "in" -> [w68]
      tunnel: w59 -> [w66]
      shift-right: [w64] -> w57
      shift-left: w58 -> [w65]
      stop <- w63 stop-if-true
      n27 = Look In Map(map=w69, key=w68) -> (value=w67:T1[])  [unwired: 1 in, 1 out]
      n28 = for {
        tunnel: w67 -> [w81] mode=indexing
        tunnel: w66 -> [w80]
        shift-right: [w72] -> w64
        shift-left: w65 -> [w75]
        tunnel: [w76] -> w63
        tunnel: [w71] -> w62
        stop <- w70 stop-if-true
        n29 = Unbundle By Name(w81) -> ("Op"=w79:T2, "Variable"=w77:T3, "Value"=w78:i32, "Result"=w74:string)
        n30 = case shown="\"TRUE\"" w79 {
          tunnel: w80 -> [_ w87 w92 w97 w102]
          tunnel: w77 -> [_ w86 w91 w96 w101]
          tunnel: w78 -> [_ w84 w89 w94 w99]
          tunnel: [TRUE w83 w88 w93 w98] -> w73
          frame "TRUE" {
          }
          frame "<" {
            n31 = Index Array(array=w87, index=w86) -> (element=w85:i32)
            n32 = Less?(x=w85, y=w84) -> (x < y?=w83:bool)
          }
          frame ">" {
            n33 = Index Array(array=w92, index=w91) -> (element=w90:i32)
            n34 = Greater?(x=w90, y=w89) -> (0:w88:bool)
          }
          frame "<=" {
            n35 = Index Array(array=w97, index=w96) -> (element=w95:i32)
            n36 = Less Or Equal?(x=w95, y=w94) -> (x <= y?=w93:bool)
          }
          frame ">=" {
            n37 = Index Array(array=w102, index=w101) -> (element=w100:i32)
            n38 = Greater Or Equal?(x=w100, y=w99) -> (x >= y?=w98:bool)
          }
        }
        n39 = case shown="True" w73 {
          tunnel: [FALSE w113] -> w76
          tunnel: w80 -> [_ w109]
          tunnel: w75 -> [w104 w111]
          tunnel: w74 -> [_ w112]
          tunnel: [w104 w110] -> w72
          tunnel: ["" w108] -> w71
          tunnel: [FALSE w107] -> w70
          frame False {
            # "OP False"
          }
          frame True {
            # "Op True"
            n40 = case shown="\"A\"" w112 {
              selector: w112 -> [w114 w118 w124]
              tunnel: [w115 w117 FALSE] -> w113
              tunnel: w111 -> [w116 w121 w125]
              tunnel: [w116 w120 w125] -> w110
              tunnel: w109 -> [_ w119 _]
              tunnel: [w114 w118 w124] -> w108
              tunnel: [w115 w117 TRUE] -> w107
              frame "R" {
                w115 = TRUE
                # "Reject Result"
              }
              frame "A" {
                w117 = TRUE
                # "Accept Part"
                n41 = Build Array (concatenate)(w121, w119) -> (w120:i32[][])
              }
              frame Default {
                # "Do a different process"
              }
            }
          }
        }
      }
    }
  }
  "Accept Array" <- w3
  n42 = Add Array Elements(numeric array=w3) -> (sum=→"Answer":i32)
